vi "generatepockelscellarray for fast z.vi"(10 "interpolated pockels cell data":dbl[](array[numeric]), 11 "piezo control":dbl[](graph)) -> (3 "pockelscellarray":dbl[](array[numeric]))   [LabVIEW 2017]
doc: "SciScan 1.2 160622"
uses:
  GFG/GFGnumericGet.vi
  GFG/GFG library.lvlib
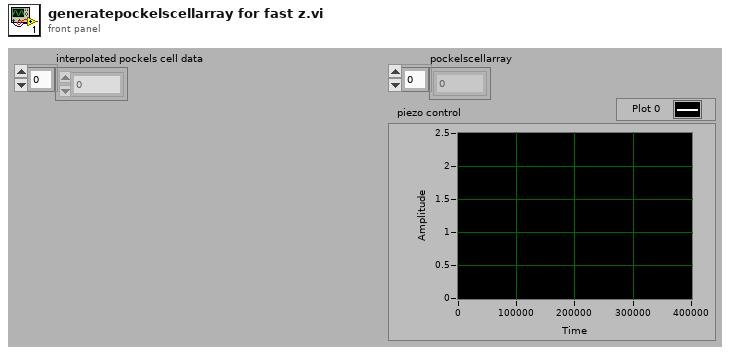
[diagram p1: front panel]
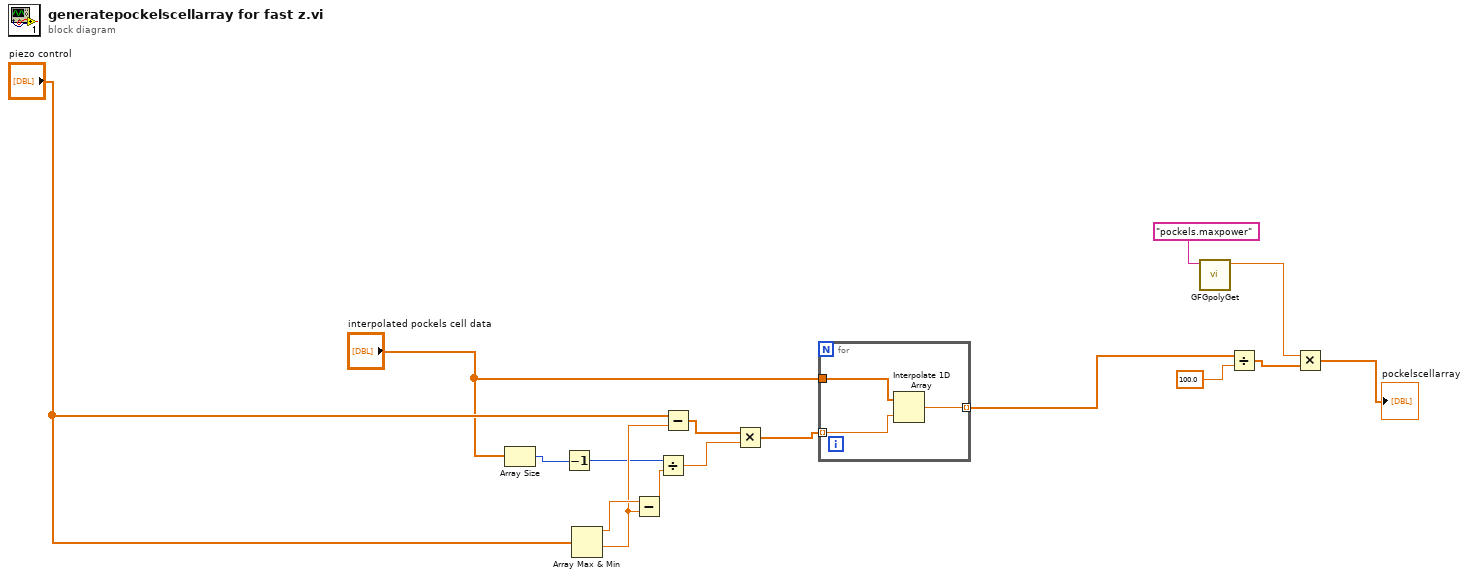
[diagram p0: block diagram]
diagram:
  n1 = Array Size(array="interpolated pockels cell data") -> (size(s)=w15:i32)
  n2 = Decrement(x=w15) -> (x-1=w1:i32)
  n3 = Array Max & Min(array="piezo control") -> (max value=w13:dbl, min value=w10:dbl)  [unwired: 2 out]
  n4 = Subtract(x=w13, y=w10) -> (x-y=w12:dbl)
  n5 = Divide(x=w1, y=w12) -> (x/y=w14:dbl)
  n6 = Subtract(x="piezo control", y=w10) -> (x-y=w11:dbl[])
  n7 = Multiply(x=w11, y=w14) -> (x*y=w9:dbl[])
  n8 = for {
    tunnel: "interpolated pockels cell data" -> [w19]
    tunnel: [w18] -> w6 mode=indexing
    tunnel: w9 -> [w17] mode=indexing
    n9 = Interpolate 1D Array(1:w17, 2:w19) -> (0:w18:dbl)
  }
  n10 = call-poly "GFGpolyGet.vi"("Variable Name in"="pockels.maxpower") -> ("Numeric"=w2:dbl)  [unwired: 8 in, 2 out]
  n11 = Divide(x=w6, y=100.0 ("x")) -> (x/y=w7:dbl[])
  n12 = Multiply(x=w2, y=w7) -> (x*y=→"pockelscellarray":dbl[])
